vi "VerifLevel.vi"(8 "error in (no error)":errorcluster, 11 "Log in":refnum<class "Log.lvclass">) -> (0 "error out":errorcluster, 2 "logging":bool, 3 "Log out":refnum<class "Log.lvclass">)   [LabVIEW 2018, in "Log.lvclass"]
uses:
  Log.lvclass
  Log.lvclass/Log.ctl
panel:
  # "T = do log"
  # "F = do not log"
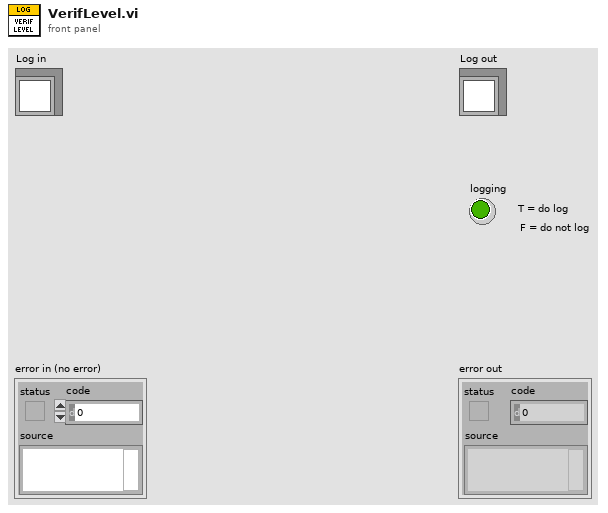
[diagram p1: front panel]
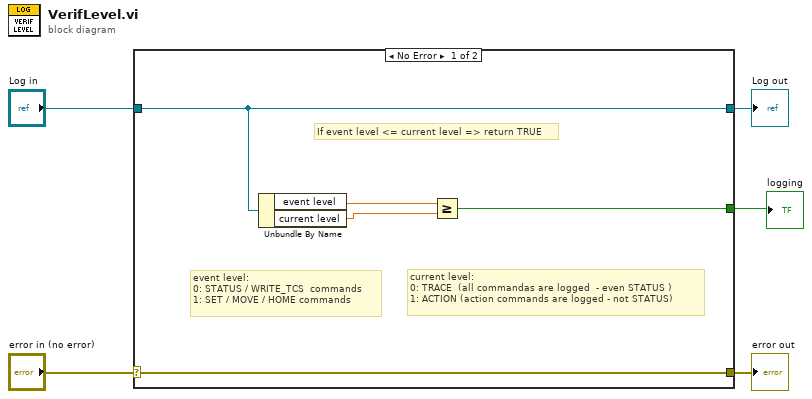
[diagram p0: block diagram]
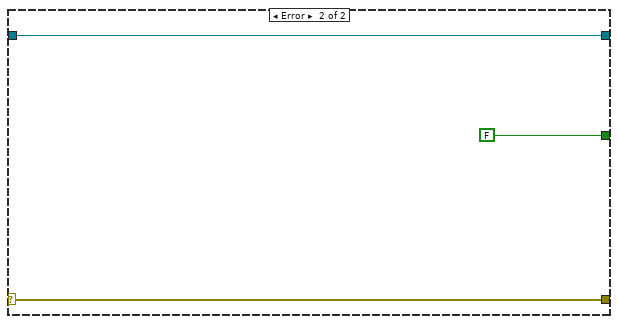
[diagram p2: hidden frame]
diagram:
  n1 = case shown="No Error" "error in (no error)" {
    selector: "error in (no error)" -> [w10 w13]
    tunnel: [w10 w13] -> w4
    tunnel: [w9 w12] -> w2
    tunnel: "Log in" -> [w9 w12]
    tunnel: [w7 FALSE] -> w1
    frame No Error {
      # "event level:\n0: STATUS / WRITE_TCS  commands\n1: SET / MOVE / HOME commands"
      # "current level:\n0: TRACE  (all commandas are logged  - even STATUS )\n1: ACTION (action commands are logged - not STATUS)"
      # "If event level <= current level => return TRUE"
      n2 = Unbundle By Name(w9) -> ("event level"=w6:dbl, "current level"=w8:dbl)
      n3 = Greater Or Equal?(x=w6, y=w8) -> (x >= y?=w7:bool)
    }
    frame Error {
    }
  }
  "error out" <- w4
  "Log out" <- w2
  "logging" <- w1
